vi "channel properties.vi"(8 "error in":errorcluster, 11 "channel in":refnum<class "TBM channel.lvclass">) -> (0 "error out":errorcluster, 2 "properties":string[](array[string]), 3 "channel out":refnum<class "TBM channel.lvclass">)   [LabVIEW 2013, in "TBM channel.lvclass"]
uses:
  TBM channel.lvclass
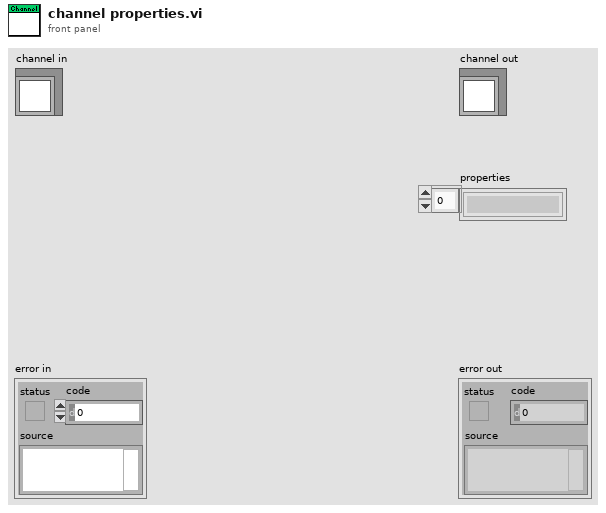
[diagram p1: front panel]
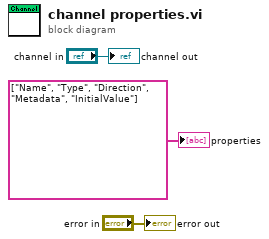
[diagram p0: block diagram]
diagram:
  "error out" <- "error in"
  "channel out" <- "channel in"
  "properties" <- string[] ["Name", "Type", "Direction", "Metadata", "InitialValue"] ("properties")
